vi "Timer.vi"(8 "error in (no error)":errorcluster, 10 "Action":enum16{"Stop", "Start", ""}(ring)=enum."Start", 11 "Cache Manager DVR in":refnum<class "Cache Manager.lvclass">) -> (0 "error out":errorcluster, 2 "Elapsed time (ms)":u32, 3 "Cache Manager DVR out":refnum<class "Cache Manager.lvclass">)   [LabVIEW 2020, in "Cache Manager.lvclass"]
uses:
  Cache Manager.lvclass
  Cache Manager.lvclass/Cache Manager.ctl
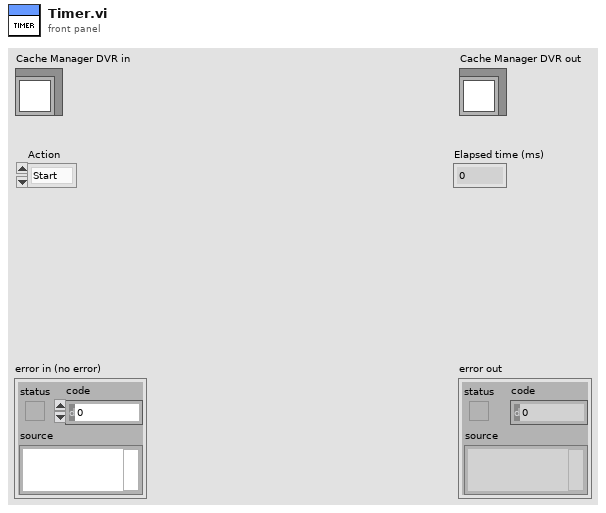
[diagram p1: front panel]
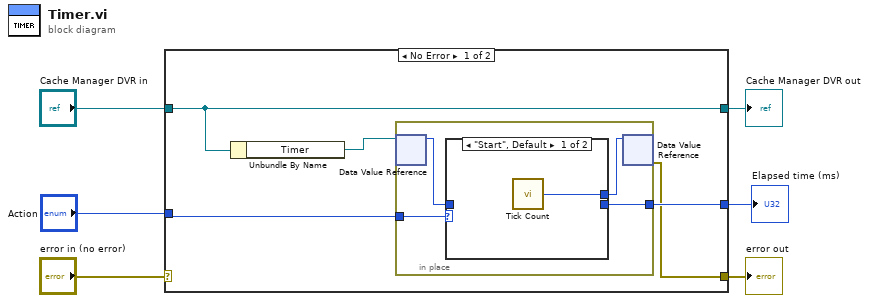
[diagram p0: block diagram]
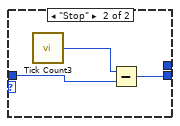
[diagram p2: hidden frame]
diagram:
  n1 = case shown="No Error" "error in (no error)" {
    selector: "error in (no error)" -> [_ w21]
    tunnel: [w7 w21] -> w5
    tunnel: [w11 w20] -> w3
    tunnel: "Cache Manager DVR in" -> [w11 w20]
    tunnel: "Action" -> [w9 _]
    tunnel: [w8 _] -> w1
    frame No Error {
      n2 = Unbundle By Name(w11) -> ("Timer"=w10:refnum<data-value>)
      n3 = in-place "In Place Element Structure" {
        in-place-border: w9 -> [w15]
        in-place-border: [w13] -> w8
        n4 = in-place-dvr #1(w10) -> (w14:u32)  [unwired: 1 out]
        n5 = case shown="\"Start\", Default" w15 {
          tunnel: w14 -> [_ w18]
          tunnel: [_ w17] -> w13
          tunnel: [w16 _] -> w12
          frame "Start", Default {
            n6 = call "Tick Count"() -> ("Tick Count(uSec)"=w16:u32)
          }
          frame "Stop" {
            n7 = call "Tick Count3"() -> ("Tick Count(uSec)"=w19:u32)
            n8 = Subtract(x=w19, y=w18) -> (x-y=w17:u32)
          }
        }
        n9 = in-place-dvr #1(w12) -> (w7:errorcluster)  [unwired: 1 out]
      }
    }
    frame Error {
    }
  }
  "error out" <- w5
  "Cache Manager DVR out" <- w3
  "Elapsed time (ms)" <- w1
